vi "SetDefinition.vi"(8 "error in (no error)":errorcluster, 10 "Definition":string[](array[string]), 11 "DefinitionList in":refnum<class "DefinitionList.lvclass">) -> (0 "error out":errorcluster, 3 "DefinitionList out":refnum<class "DefinitionList.lvclass">)   [LabVIEW 2021, in "LvMarkdown.lvlib" / "DefinitionList.lvclass"]
uses:
  DefinitionList.lvclass
  DefinitionList.lvclass/DefinitionList.ctl
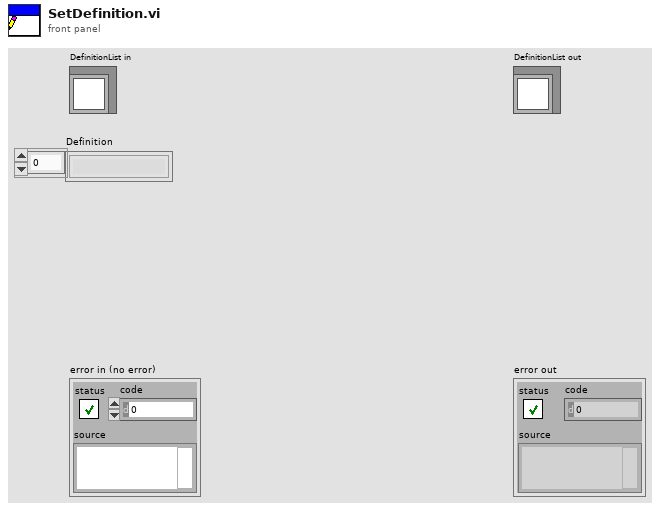
[diagram p1: front panel]
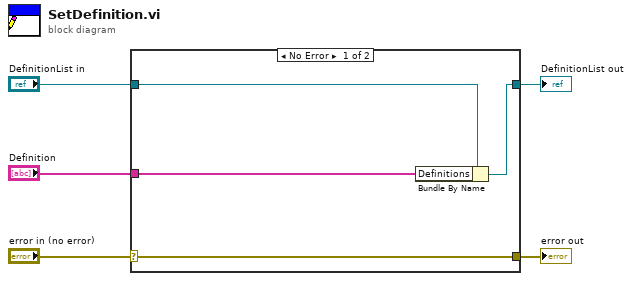
[diagram p0: block diagram]
diagram:
  n1 = case shown="No Error" "error in (no error)" {
    selector: "error in (no error)" -> [w9 w10]
    tunnel: [w9 w10] -> w4
    tunnel: [w7 w11] -> w2
    tunnel: "DefinitionList in" -> [w8 w11]
    tunnel: "Definition" -> [w6 _]
    frame No Error {
      n2 = Bundle By Name(cluster=w8, "Definitions"=w6) -> (w7:refnum<class "DefinitionList.lvclass">)
    }
    frame Error {
    }
  }
  "error out" <- w4
  "DefinitionList out" <- w2
